vi "Unload.vi"(8 "error in":errorcluster, 11 "SyringeTool in":refnum<class "SyringeTool Class.lvclass">) -> (0 "error out":errorcluster, 3 "Gantry out":refnum<class "Gantry Class.lvclass">)   [LabVIEW 2011, in "SyringeTool Class.lvclass"]
uses:
  SyringeTool Class.lvclass
  Gantry Class/Gantry Class.lvclass
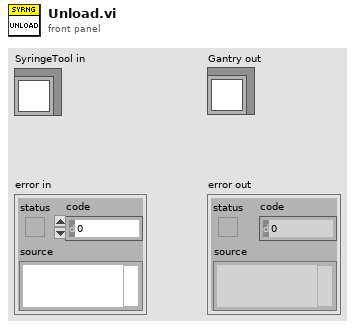
[diagram p1: front panel]
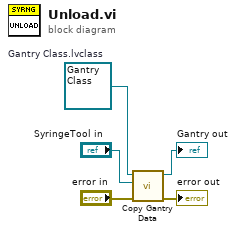
[diagram p0: block diagram]
diagram:
  w5 = refnum<class "Gantry Class.lvclass"> refnum  # Gantry Class.lvclass
  n1 = call "Copy Gantry Data.vi"("error in"="error in", "Gantry Source"="SyringeTool in", "Gantry Dest"=w5) -> ("error out"=→"error out":errorcluster, "Gantry Result"=→"Gantry out":refnum<class "Gantry Class.lvclass">)  [unwired: 7 in]
